vi "Cleanup.vi"(8 "error in (no error)":errorcluster, 11 "App in":refnum<class "App.lvclass">) -> (0 "error out":errorcluster)   [LabVIEW 2022 SP3, in "VMR-Deck.lvlib" / "App.lvclass"]
uses:
  App.lvclass
  App.lvclass/App.ctl
  WebServer/WebServer.lvclass
  VMR/VMR.lvclass
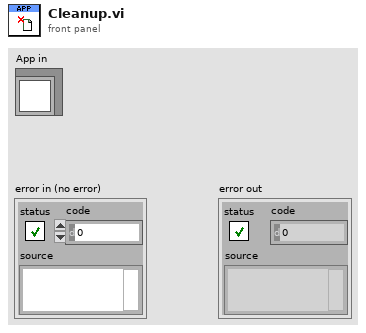
[diagram p1: front panel]
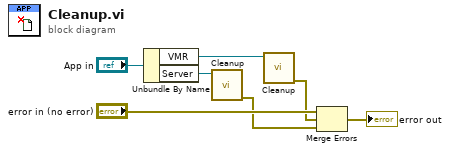
[diagram p0: block diagram]
diagram:
  n1 = Unbundle By Name("App in") -> ("VMR"=w4:refnum<class "VMR.lvclass">, "Server"=w5:refnum<class "WebServer.lvclass">)
  n2 = call "Cleanup.vi"("WebServer in"=w5) -> ("error out"=w1:errorcluster)  [unwired: 10 in]
  n3 = call "Cleanup.vi"("VMR in"=w4) -> ("error out"=w2:errorcluster)  [unwired: 10 in]
  n4 = Merge Errors("error in (no error)", w2, w1) -> (→"error out":errorcluster)
